vi "Get Base URL.vi"(8 "Error In":errorcluster, 11 "XBMC Ref":T1) -> (0 "Error Out":errorcluster, 2 "XBMC JSON Base URL":string, 3 "XBMC Ref":T1)   [LabVIEW 2013, in "LMH-Kodi.lvlib"]
uses:
  LMH-Kodi.lvlib
  Type Defs/XBMC Ref.ctl
  <vilib>/httpClient/ClientHandle.ctl
  <vilib>/httpClient/LabVIEWHTTPClient.lvlib
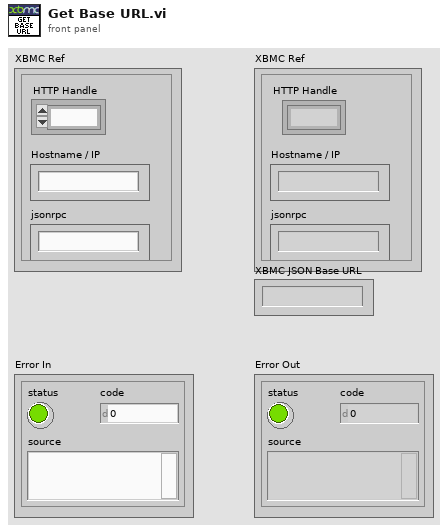
[diagram p1: front panel]
types:
  T1 = typedef "LMH-Kodi.lvlib/XBMC Ref.ctl" = cluster{"HTTP Handle":T2, "Hostname / IP":string, "jsonrpc":string}
  T2 = typedef "LabVIEWHTTPClient.lvlib/ClientHandle.ctl" = refnum<k1>
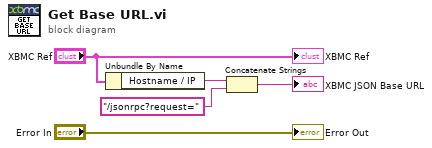
[diagram p0: block diagram]
diagram:
  n1 = Unbundle By Name("XBMC Ref") -> ("Hostname / IP"=w4:string)
  n2 = Concatenate Strings(w4, "/jsonrpc?request=" ("string")) -> (→"XBMC JSON Base URL":string)
  "XBMC Ref" <- "XBMC Ref"
  "Error Out" <- "Error In"
